vi "setName.vi"(8 "error in (no error)":errorcluster, 10 "name":string, 11 "DDSOutput in":refnum<class "DDSOutput.lvclass">) -> (0 "error out":errorcluster, 3 "DDSOutput out":refnum<class "DDSOutput.lvclass">)   [LabVIEW 2009, in "Hardware.lvlib" / "Channels.lvlib" / "DDSOutput.lvclass"]
uses:
  DDSOutput.lvclass
  DDSOutput.lvclass/DDSOutput.ctl
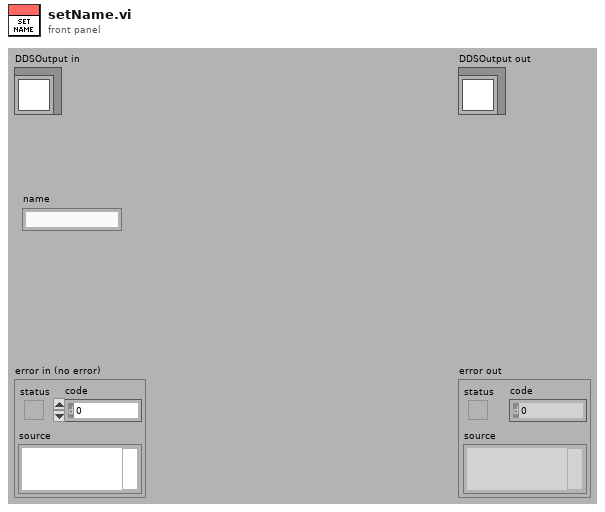
[diagram p1: front panel]
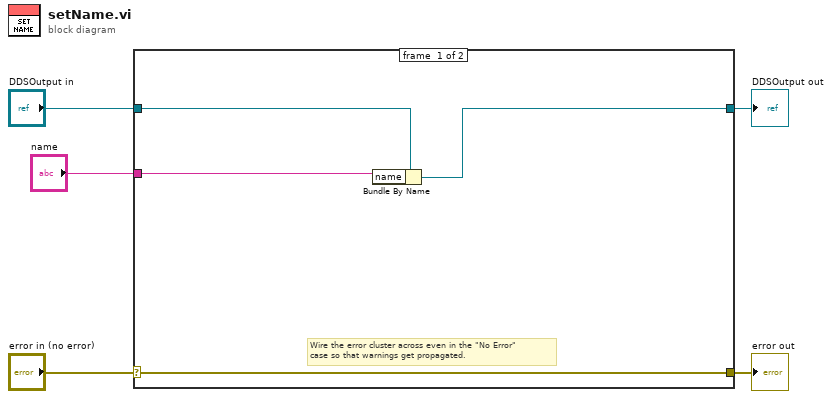
[diagram p0: block diagram]
diagram:
  n1 = case shown="No Error" "error in (no error)" {
    selector: "error in (no error)" -> [w9 w11]
    tunnel: [w9 w11] -> w4
    tunnel: [w7 w10] -> w2
    tunnel: "DDSOutput in" -> [w8 w10]
    tunnel: "name" -> [w6 _]
    frame #0 {
      # "Wire the error cluster across even in the \"No Error\"\ncase so that warnings get propagated."
      n2 = Bundle By Name(cluster=w8, "name"=w6) -> (w7:refnum<class "DDSOutput.lvclass">)
    }
    frame #1 {
    }
  }
  "error out" <- w4
  "DDSOutput out" <- w2
